vi "Create From Variant.vi"(8 "error in (no error)":errorcluster, 10 "Variant":variant, 11 "JSON String in":refnum<class "JSON String.lvclass">) -> (0 "error out":errorcluster, 3 "JSON String out":refnum<class "JSON String.lvclass">)   [LabVIEW 2015, in "LVJSON.lvlib" / "JSON String.lvclass"]
uses:
  JSON String.lvclass
  JSON String.lvclass/JSON String.ctl
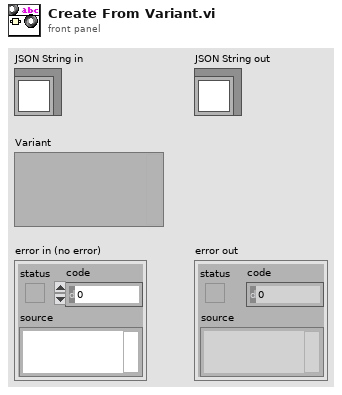
[diagram p1: front panel]
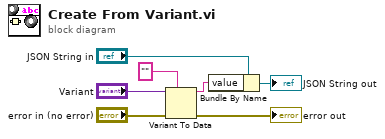
[diagram p0: block diagram]
diagram:
  n1 = Variant To Data(error in="error in (no error)", type="", Variant="Variant") -> (data=w3:string, error out=→"error out":errorcluster)
  n2 = Bundle By Name(cluster="JSON String in", "value"=w3) -> (→"JSON String out":refnum<class "JSON String.lvclass">)
